vi "Password.vi"() -> (2 "验证成功？":bool)   [LabVIEW 2018]
panel:
  in  "取消按钮":bool
  in  "确定按钮":bool
  in  "管理员口令":string
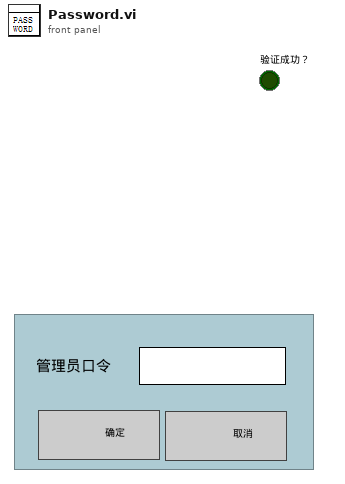
[diagram p1: front panel]
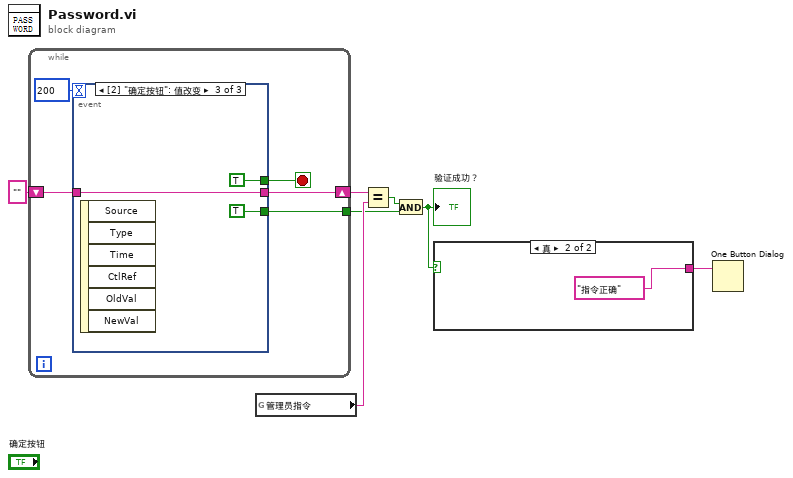
[diagram p0: block diagram]
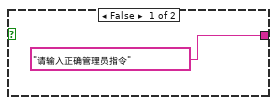
[diagram p2: hidden frame]
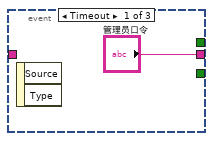
[diagram p3: hidden frame]
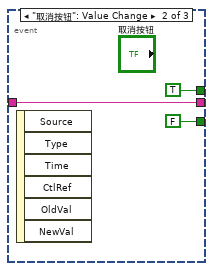
[diagram p4: hidden frame]
diagram:
  n1 = while {
    shift-right: [w12] -> w6
    shift-left: "" ("管理员口令") -> [w10]
    tunnel: [w9] -> w3
    stop <- w11 stop-if-true
    n2 = event shown="[2] \"确定按钮\": 值改变" {
      selector: _ -> [_ _ _]
      dyn-events: _ -> [_ _ _]
      timeout: 200 -> [_ _ _]
      tunnel: ["管理员口令" w15 w18] -> w12
      tunnel: [_ TRUE TRUE] -> w11
      tunnel: w10 -> [_ w15 w18]
      tunnel: [_ FALSE TRUE] -> w9
      event Timeout {
        n3 = event-data() -> ()  [unwired: 1 in, 2 out]
      }
      event "取消按钮": Value Change {
        n4 = event-data() -> ()  [unwired: 1 in, 6 out]
      }
      event "确定按钮": Value Change {
        n5 = event-data() -> ()  [unwired: 1 in, 6 out]
      }
    }
  }
  n6 = global read "消息通知.vi" "管理员指令"() -> (w5:string)
  n7 = Equal?(x=w6, y=w5) -> (x = y?=w4:bool)
  n8 = And(x=w4, y=w3) -> (x .and. y?=w2:bool)
  "验证成功？" <- w2
  n9 = case shown="真" w2 {
    tunnel: ["请输入正确管理员指令" ("消息") "指令正确" ("消息")] -> w1
    frame False {
    }
    frame True {
    }
  }
  n10 = One Button Dialog(message=w1) -> ()  [unwired: 1 in, 1 out]
